vi "Open Hardware.vi"(8 "error in (no error)":errorcluster, 11 "Instrument.VRM in":refnum<class "Instrument.OxfordVRM.lvclass">) -> (0 "error out":errorcluster, 3 "Instrument.VRM out":refnum<class "Instrument.OxfordVRM.lvclass">)   [LabVIEW 2019, in "Instrument.OxfordVRM.lvclass"]
uses:
  Instrument.OxfordVRM.lvclass
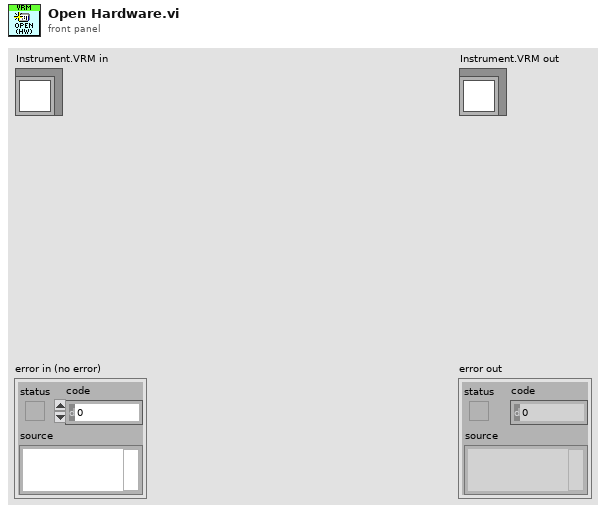
[diagram p1: front panel]
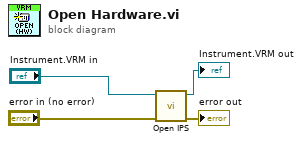
[diagram p0: block diagram]
diagram:
  n1 = call "Open IPS.vi"("error in (no error)"="error in (no error)", "Instrument.OxfordVRM in"="Instrument.VRM in") -> ("error out"=→"error out":errorcluster, "Instrument.OxfordVRM out"=→"Instrument.VRM out":refnum<class "Instrument.OxfordVRM.lvclass">)  [unwired: 8 in]
